vi "IPS120 RH1 - Get Status.vi"(1 "GPIB Address":string="1:25") -> (0 "Magnet Status":T1={"Sweep Status"=enum."To Zero", "Leads Current (A)"=0.0, "Leads Voltage (V)"=-0.02, "Leads Field (T)"=0.0, "Switch Heater"=FALSE, "Setpoint (A)"=0.0, "Sweep Rate (A/min)"=0.0, "System Status"=enum."Normal", "Limit Status"=enum."Normal", "Persistent Current (A)"=0.0, "Control Status"=FALSE, "Persistent Field (T)"=0.0} {"Leads Field (T)" format="%.3f"; "Persistent Field (T)" format="%.3f"; "Persistent Current (A)" format="%.3f"; "Setpoint (A)" format="%.3f"; "Leads Voltage (V)" format="%.2f"; "Sweep Rate (A/min)" format="%.2f"; "Leads Current (A)" format="%.3f"})   [LabVIEW 2019]
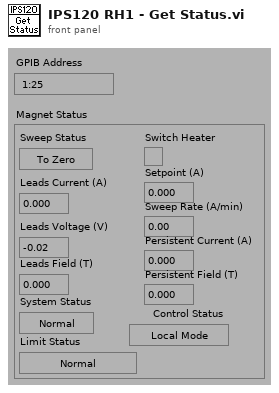
[diagram p1: front panel]
types:
  T1 = cluster{"Sweep Status":enum16{"Hold", "To Setpoint", "To Zero", "Clamped"}, "Leads Current (A)":dbl, "Leads Voltage (V)":dbl, "Leads Field (T)":dbl, "Switch Heater":bool, "Setpoint (A)":dbl, "Sweep Rate (A/min)":dbl, "System Status":enum16{"Normal", "Quenched", "Over Heated", "Warming Up"}, "Limit Status":enum16{"Normal", "Positive Voltage Limit", "Negative Voltage Limit", "Negative Current Limit", "Positive Current Limit"}, "Persistent Current (A)":dbl, "Control Status":bool, "Persistent Field (T)":dbl}
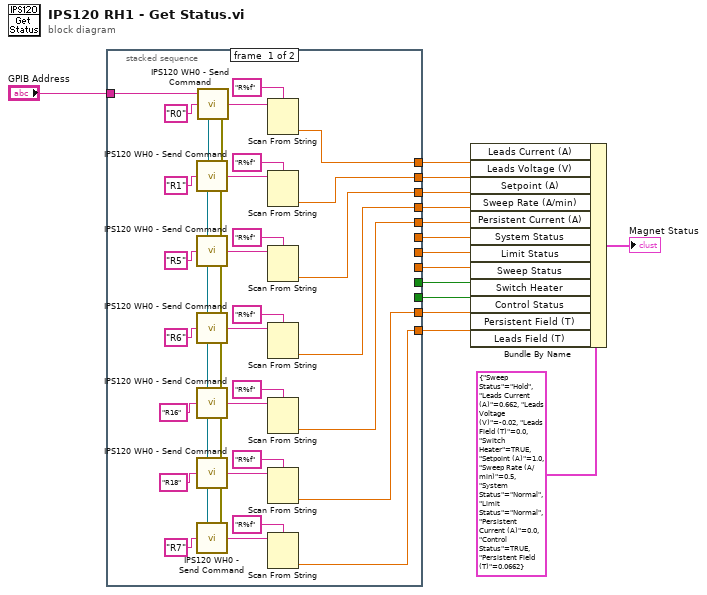
[diagram p0: block diagram]
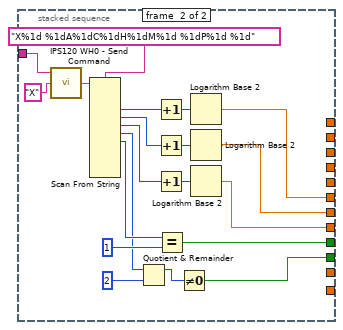
[diagram p2: hidden frame]
diagram:
  n1 = stacked-sequence {
    tunnel: "GPIB Address" -> [w22 w75]
    tunnel: [w56 _] -> w11
    tunnel: [w53 _] -> w12
    tunnel: [w52 _] -> w13
    tunnel: [w51 _] -> w14
    tunnel: [w44 _] -> w15
    tunnel: [_ w70] -> w9
    tunnel: [_ w62] -> w8
    tunnel: [_ w63] -> w7
    tunnel: [_ w64] -> w6
    tunnel: [_ w58] -> w5
    tunnel: [w33 _] -> w4
    tunnel: [w29 _] -> w1
    frame #0 {
      n2 = call "IPS120 WH0 - Send Command.vi"("Command String"="R0", "VISA Address"=w22) -> ("error out"=w28:errorcluster, "Response String"=w43:string, "VISA resource name out"=w21:refnum<visa-resource-name>)  [unwired: 1 in]
      n3 = call "IPS120 WH0 - Send Command.vi"("error in (no error)"=w28, "Command String"="R1", "VISA Address"=w21) -> ("error out"=w27:errorcluster, "Response String"=w48:string, "VISA resource name out"=w20:refnum<visa-resource-name>)
      n4 = call "IPS120 WH0 - Send Command.vi"("error in (no error)"=w27, "Command String"="R5", "VISA Address"=w20) -> ("error out"=w26:errorcluster, "Response String"=w49:string, "VISA resource name out"=w19:refnum<visa-resource-name>)
      n5 = call "IPS120 WH0 - Send Command.vi"("error in (no error)"=w26, "Command String"="R6", "VISA Address"=w19) -> ("error out"=w25:errorcluster, "Response String"=w50:string, "VISA resource name out"=w18:refnum<visa-resource-name>)
      n6 = call "IPS120 WH0 - Send Command.vi"("error in (no error)"=w25, "Command String"="R16", "VISA Address"=w18) -> ("error out"=w24:errorcluster, "Response String"=w55:string, "VISA resource name out"=w17:refnum<visa-resource-name>)
      n7 = call "IPS120 WH0 - Send Command.vi"("error in (no error)"=w24, "Command String"="R18", "VISA Address"=w17) -> ("error out"=w23:errorcluster, "Response String"=w34:string, "VISA resource name out"=w16:refnum<visa-resource-name>)
      n8 = call "IPS120 WH0 - Send Command.vi"("error in (no error)"=w23, "Command String"="R7", "VISA Address"=w16) -> ("Response String"=w32:string)  [unwired: 2 out]
      n9 = Scan From String(format string="R%f", input string=w43) -> (output 1=w44:dbl)  [unwired: 3 in, 3 out]
      n10 = Scan From String(format string="R%f", input string=w48) -> (output 1=w51:dbl)  [unwired: 3 in, 3 out]
      n11 = Scan From String(format string="R%f", input string=w49) -> (output 1=w52:dbl)  [unwired: 3 in, 3 out]
      n12 = Scan From String(format string="R%f", input string=w50) -> (output 1=w53:dbl)  [unwired: 3 in, 3 out]
      n13 = Scan From String(format string="R%f", input string=w55) -> (output 1=w56:dbl)  [unwired: 3 in, 3 out]
      n14 = Scan From String(format string="R%f", input string=w34) -> (output 1=w33:dbl)  [unwired: 3 in, 3 out]
      n15 = Scan From String(format string="R%f", input string=w32) -> (output 1=w29:dbl)  [unwired: 3 in, 3 out]
    }
    frame #1 {
      n16 = call "IPS120 WH0 - Send Command.vi"("Command String"="X", "VISA Address"=w75) -> ("Response String"=w73:string)  [unwired: 1 in, 2 out]
      n17 = Scan From String(format string="X%1d %1dA%1dC%1dH%1dM%1d %1dP%1d %1d", input string=w73) -> (output 1=w72:i32, output 2=w67:i32, output 3=w66:i32, output 4=w60:i32, output 5=w61:i32)  [unwired: 15 in, 3 out]
      n18 = Quotient & Remainder(x=w60, y=2) -> (x-y*floor(x/y)=w57:i32)  [unwired: 1 out]
      n19 = Increment(x=w72) -> (x+1=w71:i32)
      n20 = Increment(x=w67) -> (x+1=w69:i32)
      n21 = Increment(x=w66) -> (x+1=w68:i32)
      n22 = Equal?(x=w61, y=1) -> (x = y?=w64:bool)
      n23 = Not Equal To 0?(x=w57) -> (x != 0?=w58:bool)
      n24 = Logarithm Base 2(1:w71) -> (0:w70:dbl)
      n25 = Logarithm Base 2(1:w69) -> (0:w62:dbl)
      n26 = Logarithm Base 2(1:w68) -> (0:w63:dbl)
    }
  }
  n27 = Bundle By Name(cluster=T1 {"Sweep Status"=enum."Hold", "Leads Current (A)"=0.662, "Leads Voltage (V)"=-0.02, "Leads Field (T)"=0.0, "Switch Heater"=TRUE, "Setpoint (A)"=1.0, "Sweep Rate (A/min)"=0.5, "System Status"=enum."Normal", "Limit Status"=enum."Normal", "Persistent Current (A)"=0.0, "Control Status"=TRUE, "Persistent Field (T)"=0.0662} ("Magnet Status"), "Leads Current (A)"=w15, "Leads Voltage (V)"=w14, "Setpoint (A)"=w13, "Sweep Rate (A/min)"=w12, "Persistent Current (A)"=w11, "System Status"=w9, "Limit Status"=w8, "Sweep Status"=w7, "Switch Heater"=w6, "Control Status"=w5, "Persistent Field (T)"=w4, "Leads Field (T)"=w1) -> (→"Magnet Status":T1)
